vi "Write to Target FIFO (U256).vi"(7 "Host FIFO":refnum<k21>="Target fifo u64", 8 "Input Valid":bool, 11 "Input Data":T1) -> (2 "Data Written":bool, 3 "data out":u64, 6 "Ready For Input":bool)   [LabVIEW 2012]
doc: "<b> This VI transfers U256 data to Host in U64 Chunks </b>\n\nIt takes 4 Ticks for this VI to insert data into Host FIFO if there is space available in the Host FIFO. The VI will retry sending data into Host FIFO until space is available. Further it will send \"Ready for Input\" signal to upstream block as when it can accept data."
uses:
  <vilib>/rvi/DataTransferAndStorage/Container/Common/niFpgaContainerMetaDataKey.ctl
  <vilib>/rvi/DataTransferAndStorage/Container/Common/niFpgaContainerState.ctl
  <vilib>/rvi/DataTransferAndStorage/Container/Common/niFpgaDataTypeControl.ctl
  <vilib>/rvi/DataTransferAndStorage/Container/Common/niFpgaContainerImplementationControl.ctl
  <vilib>/rvi/DataTransferAndStorage/Container/Common/niFpgaContainerArbitrationOptionsControl.ctl
  <vilib>/rvi/DataTransferAndStorage/Container/Common/niFpgaTransferTypeControl.ctl
  <vilib>/rvi/DataTransferAndStorage/Container/Common/niFpgaContainerInitializationParameters.ctl
  <vilib>/rvi/Memory/Memory_Types/niFpgaMemoryInterfaceConfiguration.ctl
  <vilib>/rvi/FIFO/Fifo_Types/niFpgaFifoControlLogicControl.ctl
  <vilib>/rvi/DataTransferAndStorage/Container/Common/niFpgaContainerGetUniqueNameForEmu.vi
  <vilib>/rvi/DataTransferAndStorage/Container/Common/niFpgaContainerSetEmuInfo.vi
  <vilib>/rvi/eio/common/nirviEmuReportErrorAndStop.vi
  <vilib>/rvi/DataTransferAndStorage/Container/Common/niFpgaContainerExecOnDevCompGetState.vi
  <vilib>/rvi/FIFO/Fifo_Resource/nirvififoEmulationSetSize.vi
  <vilib>/rvi/interface/RandomDataEmulation/nirviRandomDataFPGAFIFO.vi
  <vilib>/rvi/interface/RandomDataEmulation/niFpgaRandomDataHandleErrors.vi
  <vilib>/rvi/Emulation/niFpgaSctlEmulationGetInTimedLoop.vi
  <vilib>/rvi/Emulation/niFpgaSctlEmulationFifoFullMgr.vi
  <vilib>/rvi/errors/niFpgaSetErrorForExecOnDevCompSimple.vi
  <vilib>/rvi/Emulation/niFpgaSctlEmulationResourceMgr.vi
  <vilib>/rvi/LocalResourceManager/LocalResourceManager.xnode
  <vilib>/rvi/DataTransferAndStorage/Container/XNode/niFpgaContainer.xnode
  <vilib>/rvi/FIFO/Fifo_Resource/niFpgaFifoEmulationRefIn.vi
  <instrlib>/FlexRIO/Libraries/Helper VIs/NI FlexRIO Helper VIs.lvlib
panel:
  out "data valids written":u64
  out "data validsafter handshanke":u64
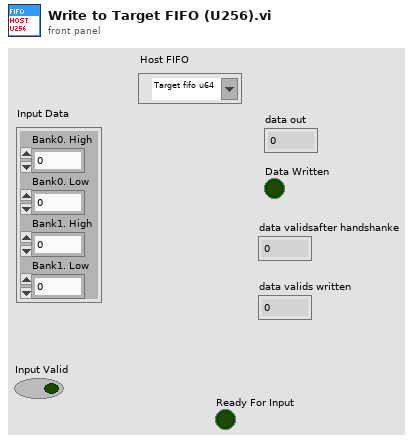
[diagram p1: front panel]
types:
  T1 = cluster{"Bank0. High":u64, "Bank0. Low":u64, "Bank1. High":u64, "Bank1. Low":u64}
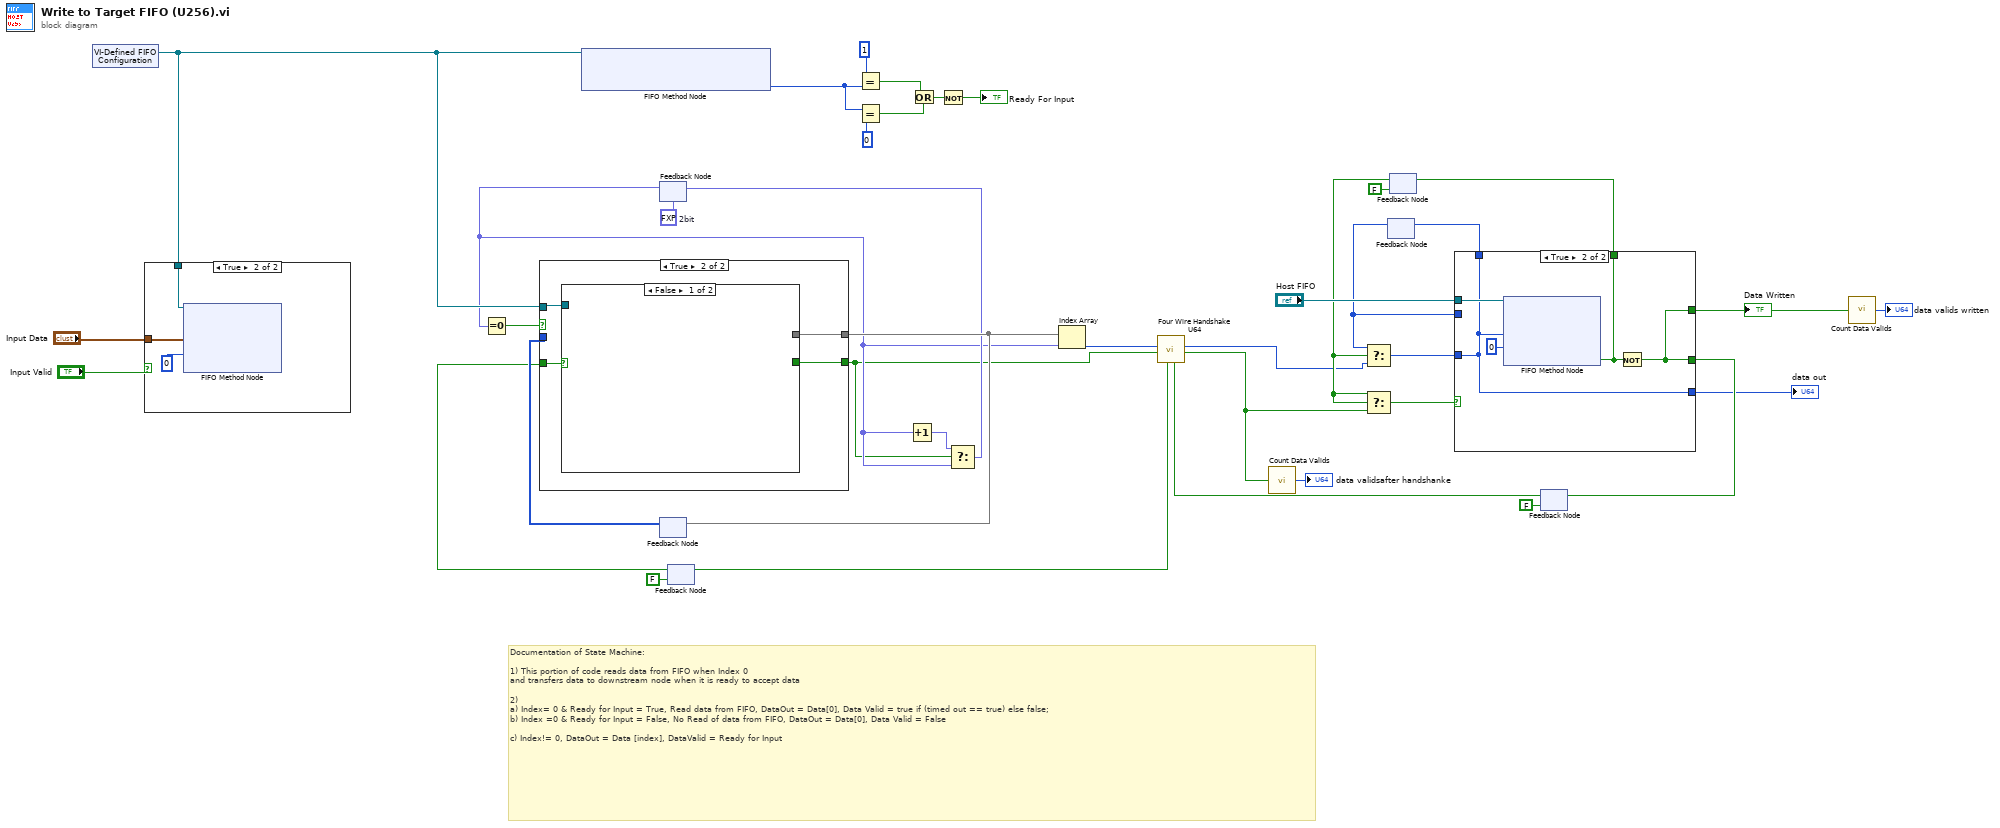
[diagram p0: block diagram]
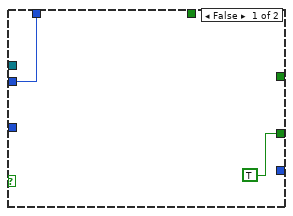
[diagram p2: hidden frame]
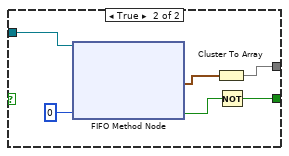
[diagram p4: hidden frame]
diagram:
  w27 = fxp<+,2,2> 0.0  # 2bit
  # "Documentation of State Machine:\n\n1) This portion of code reads data from FIFO when Index 0\nand transfers data to downstream node when it is ready to accept data\n\n2) \na) Index= 0 & Ready for Input = True, Read data from FIFO, DataOut = Data[0], Data Valid = true if (timed out == true) else false; \nb) Index =0 & Ready for Input = False, No Read of data from FIFO, DataOut = Data[0], Data Valid = False\n\nc) Index!= 0, DataOut = Data [index], DataValid = Ready for Input"
  n1 = xnode "VI-Defined FIFO Configuration"() -> ("FIFO Out"=w32:refnum<k21>)
  n2 = case shown="True" "Input Valid" {
    tunnel: w32 -> [_ w42]
    tunnel: "Input Data" -> [_ w41]
    frame False {
    }
    frame True {
      n3 = xnode ("FIFO Method Node")("Element"=w41, "Timeout"=0, "FIFO In"=w42) -> ()  [unwired: 2 out]
    }
  }
  n4 = xnode ("FIFO Method Node")("FIFO In"=w32) -> ("Number of Elements to Write"=w35:u32)  [unwired: 1 out]
  n5 = feedback #1(w27) -> (w21:fxp<+,2,2>)
  n6 = Equal To 0?(x=w21) -> (x = 0?=w25:bool)
  n7 = feedback #2() -> (w29:u64[])  [unwired: 1 in]
  n8 = feedback #3(FALSE ("ready for input")) -> (w24:bool)
  n9 = case shown="True" w25 {
    tunnel: [w43 w46] -> w18
    tunnel: w32 -> [_ w48]
    tunnel: [w44 w47] -> w28
    tunnel: w29 -> [w44 _]
    tunnel: w24 -> [w43 w45]
    frame False {
    }
    frame True {
      n10 = case shown="False" w45 {
        tunnel: w48 -> [_ w54]
        tunnel: [_ w50] -> w47
        tunnel: [_ w49] -> w46
        frame False {
        }
        frame True {
          n11 = xnode ("FIFO Method Node")("Timeout"=0, "FIFO In"=w54) -> ("Element"=w51:T1, "Timed Out?"=w53:bool)  [unwired: 1 out]
          n12 = Cluster To Array(cluster=w51) -> (array=w50:u64[])
          n13 = Not(x=w53) -> (.not. x?=w49:bool)
        }
      }
    }
  }
  n14 = feedback-in #2(w28) -> ()
  n15 = Equal?(x=u32 1 ("y"), y=w35) -> (x = y?=w37:bool)
  n16 = Equal?(x=w35, y=u32 0) -> (x = y?=w36:bool)
  n17 = Increment(x=w21) -> (x+1=w23:fxp<+,2,2>)
  n18 = Or(x=w37, y=w36) -> (x .or. y?=w39:bool)
  n19 = Not(x=w39) -> (.not. x?=→"Ready For Input":bool)
  n20 = Select(t=w23, s=w18, f=w21) -> (s? t:f=w22:fxp<+,2,2>)
  n21 = feedback-in #1(w22) -> ()
  n22 = Index Array(array=w28, index=w21) -> (element=w19:u64)
  n23 = feedback #4() -> (w1:u64)  [unwired: 1 in]
  n24 = feedback #5(FALSE ("Timed Out?")) -> (w7:bool)
  n25 = feedback #6(FALSE) -> (w14:bool)
  n26 = call <instrlib>:"Four Wire Handshake U64.vi"("ready for output"=w14, "data valid"=w18, "Data"=w19) -> ("valid out"=w6:bool, "data out"=w2:u64, "ready for input"=w16:bool)  [unwired: 5 in, 1 out]
  n27 = feedback-in #3(w16) -> ()
  n28 = call <userlib>:"Count Data Valids.vi"("Data Valid"=w6) -> ("Counter"=→"data validsafter handshanke":u64)  [unwired: 14 in]
  n29 = Select(t=w1, s=w7, f=w2) -> (s? t:f=w9:u64)
  n30 = Select(t=w7, s=w7, f=w6) -> (s? t:f=w5:bool)
  n31 = case shown="True" w5 {
    tunnel: "Host FIFO" -> [_ w61]
    tunnel: [TRUE w59] -> w12
    tunnel: [_ w59] -> w11
    tunnel: [_ w58] -> w10
    tunnel: w9 -> [_ w57]
    tunnel: [w56 w57] -> w8
    tunnel: w1 -> [w56 _]
    tunnel: [_ w57] -> w3
    frame False {
    }
    frame True {
      n32 = xnode ("FIFO Method Node")("Element"=w57, "Timeout"=0, "FIFO In"=w61) -> ("Timed Out?"=w58:bool)  [unwired: 1 out]
      n33 = Not(x=w58) -> (.not. x?=w59:bool)
    }
  }
  "data out" <- w3
  "Data Written" <- w11
  n34 = feedback-in #4(w8) -> ()
  n35 = feedback-in #5(w10) -> ()
  n36 = feedback-in #6(w12) -> ()
  n37 = call <userlib>:"Count Data Valids.vi"("Data Valid"=w11) -> ("Counter"=→"data valids written":u64)  [unwired: 14 in]
